vi "error to fault.vi"(8 "error cluster":errorcluster) -> (3 "response string":string)   [LabVIEW 2014]
doc: "Converts a LV error message to an XML-RPC fault response"
uses:
  <vilib>/Utility/error.llb/DialogType.ctl
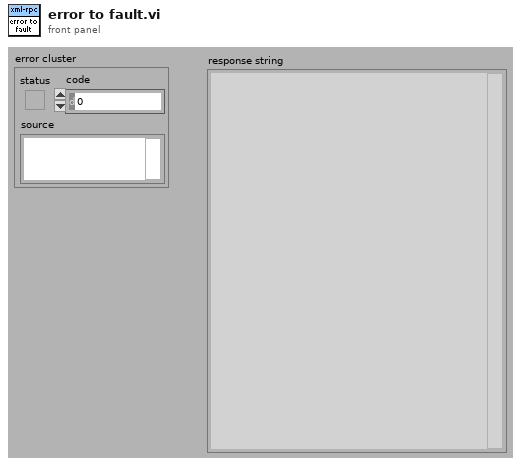
[diagram p1: front panel]
types:
  T1 = typedef "DialogType.ctl" = u16
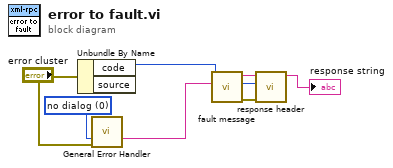
[diagram p0: block diagram]
diagram:
  w1 = T1 0 items=["no dialog", "OK message", "continue or stop message", "OK message + warnings", "continue/stop + warnings"] ("type of dialog (OK msg:1)")
  n1 = Unbundle By Name("error cluster") -> ("code"=w4:i32)  [unwired: 1 out]
  n2 = call <vilib>:"General Error Handler.vi"("type of dialog (OK msg:1)"=w1, "error in (no error)"="error cluster") -> ("message"=w2:string)  [unwired: 9 in, 4 out]
  n3 = call "fault message.vi"("faultString"=w2, "faultCode"=w4) -> ("error out"=w6:errorcluster, "length"=w8:i32, "fault string"=w7:string)  [unwired: 7 in]
  n4 = call "response header.vi"("error in"=w6, "Content-Length"=w8, "Content String"=w7) -> ("response string"=→"response string":string)  [unwired: 7 in, 1 out]
